vi "DeleteFromHandAndAddToDoor.vi"(9 "Tile":u16(ring), 10 "Player":T1) -> (2 "NewPlayer":T1)   [LabVIEW 2025]
uses:
  Controls/Player.ctl
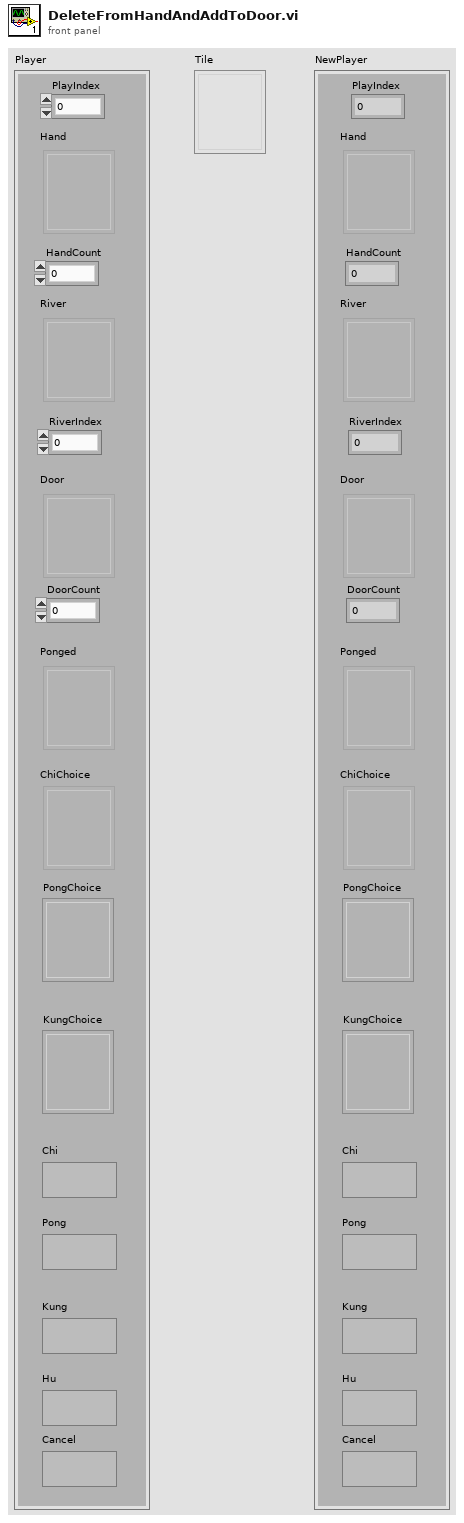
[diagram p1: front panel]
types:
  T1 = typedef "Player.ctl" = cluster{"PlayIndex":u16, "Hand":u16[], "HandCount":u16, "RiverIndex":u16, "Door":u16[], "DoorCount":u16, "Ponged":u16[], "ChiChoice":u16[][], "River":u16[][], "Chi":bool, "Pong":bool, "Kung":bool, "Hu":bool, "Cancel":bool, "PongChoice":u16, "KungChoice":u16}
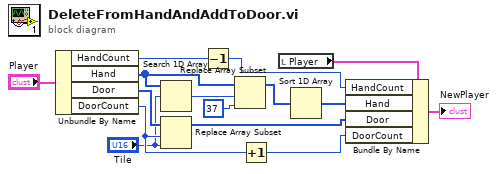
[diagram p0: block diagram]
diagram:
  n1 = Unbundle By Name("Player") -> ("HandCount"=w2:u16, "Hand"=w11:u16[], "Door"=w6:u16[], "DoorCount"=w4:u16)
  n2 = Search 1D Array(1D array=w11, element="Tile") -> (index of element=w12:i32)  [unwired: 1 in]
  n3 = Replace Array Subset(array=w6, new element="Tile", index=w4) -> (w7:u16[])
  n4 = Decrement(x=w2) -> (x-1=w1:u16)
  n5 = Replace Array Subset(array=w11, new element=37, index=w12) -> (w10:u16[])
  n6 = Increment(x=w4) -> (x+1=w5:u16)
  n7 = local read "Player"() -> (w13:T1)
  n8 = Sort 1D Array(array=w10) -> (sorted array=w9:u16[])
  n9 = Bundle By Name(cluster=w13, "HandCount"=w1, "Hand"=w9, "Door"=w7, "DoorCount"=w5) -> (→"NewPlayer":T1)
